vi "MotorCloseSynchronization.vi"(0 "error in (no error)":errorcluster, 1 "Queue Reference in":refnum<notifier>[](array[refnum]), 2 "Notifiers in":refnum<notifier>[](array[refnum]), 4 "Queue in":refnum<queue>) -> (3 "error out (no error)":errorcluster caption="error out")   [LabVIEW 2009]
uses:
  Controls/MotorCommand.ctl
  Controls/MotorCommandBasic.ctl
  Controls/MotorStatus.ctl
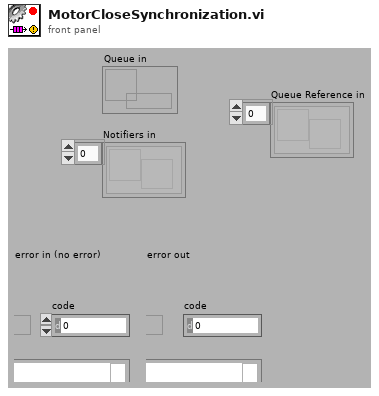
[diagram p1: front panel]
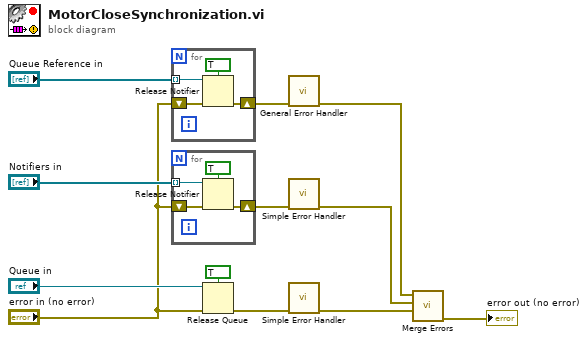
[diagram p0: block diagram]
diagram:
  n1 = for {
    shift-right: [w13] -> w6
    shift-left: "error in (no error)" -> [w16]
    tunnel: "Queue Reference in" -> [w14] mode=indexing
    n2 = Release Notifier(notifier=w14, force destroy? (F)=TRUE ("forcer la destruction ? (F)"), error in (no error)=w16) -> (error out=w13:errorcluster)  [unwired: 2 out]
  }
  n3 = for {
    tunnel: "Notifiers in" -> [w18] mode=indexing
    shift-right: [w17] -> w4
    shift-left: "error in (no error)" -> [w20]
    n4 = Release Notifier(notifier=w18, force destroy? (F)=TRUE ("forcer la destruction ? (F)"), error in (no error)=w20) -> (error out=w17:errorcluster)  [unwired: 2 out]
  }
  n5 = Release Queue(queue="Queue in", force destroy? (F)=TRUE ("forcer la destruction ? (F)"), error in (no error)="error in (no error)") -> (error out=w2:errorcluster)  [unwired: 2 out]
  n6 = call <vilib>:"General Error Handler.vi"("error in (no error)"=w6) -> ("error out"=w5:errorcluster)  [unwired: 1 in, 13 out]
  n7 = call <vilib>:"Simple Error Handler.vi"("error in (no error)"=w4) -> ("error out"=w3:errorcluster)  [unwired: 1 in, 7 out]
  n8 = call <vilib>:"Simple Error Handler.vi"("error in (no error)"=w2) -> ("error out"=w1:errorcluster)  [unwired: 1 in, 7 out]
  n9 = call <vilib>:"Merge Errors.vi"("error in 3 (no error)"=w1, "error in 2 (no error)"=w3, "error in 1 (no error)"=w5) -> ("error out"=→"error out (no error)":errorcluster)  [unwired: 1 in, 3 out]
